vi "find_preamble2x1.vi"(0 "received \ntime symbol":cdb[](array[numeric]), 5 "FFT Size":u32, 7 "CP Length":u32, 9 "1st preamble":cdb[](array[numeric]), 11 "2nd preamble":cdb[](array[numeric])) -> (4 "OFDM Symbol":cdb[](array[numeric]))   [LabVIEW 2020]
uses:
  <vilib>/Analysis/2dsp.llb/Complex FFT.vi
  <vilib>/Analysis/baseanly.llb/Complex A x B.vi
  <vilib>/Analysis/NI_AALBase.lvlib
  <vilib>/Analysis/NI_AALPro.lvlib
panel:
  out "Waveform Chart 4":dbl[](graph)
  out "size(s)":i32
  out "Array":i32[](array[numeric])
  out "Waveform Chart 3":dbl[](graph)
  out "Channel Estimation":cdb[][](array[numeric])
  out "x-y":i32
  out "Waveform Chart 2":dbl[](graph)
  out "Waveform Chart":dbl[](graph)
  out "max value 2":dbl
  out "max value":dbl
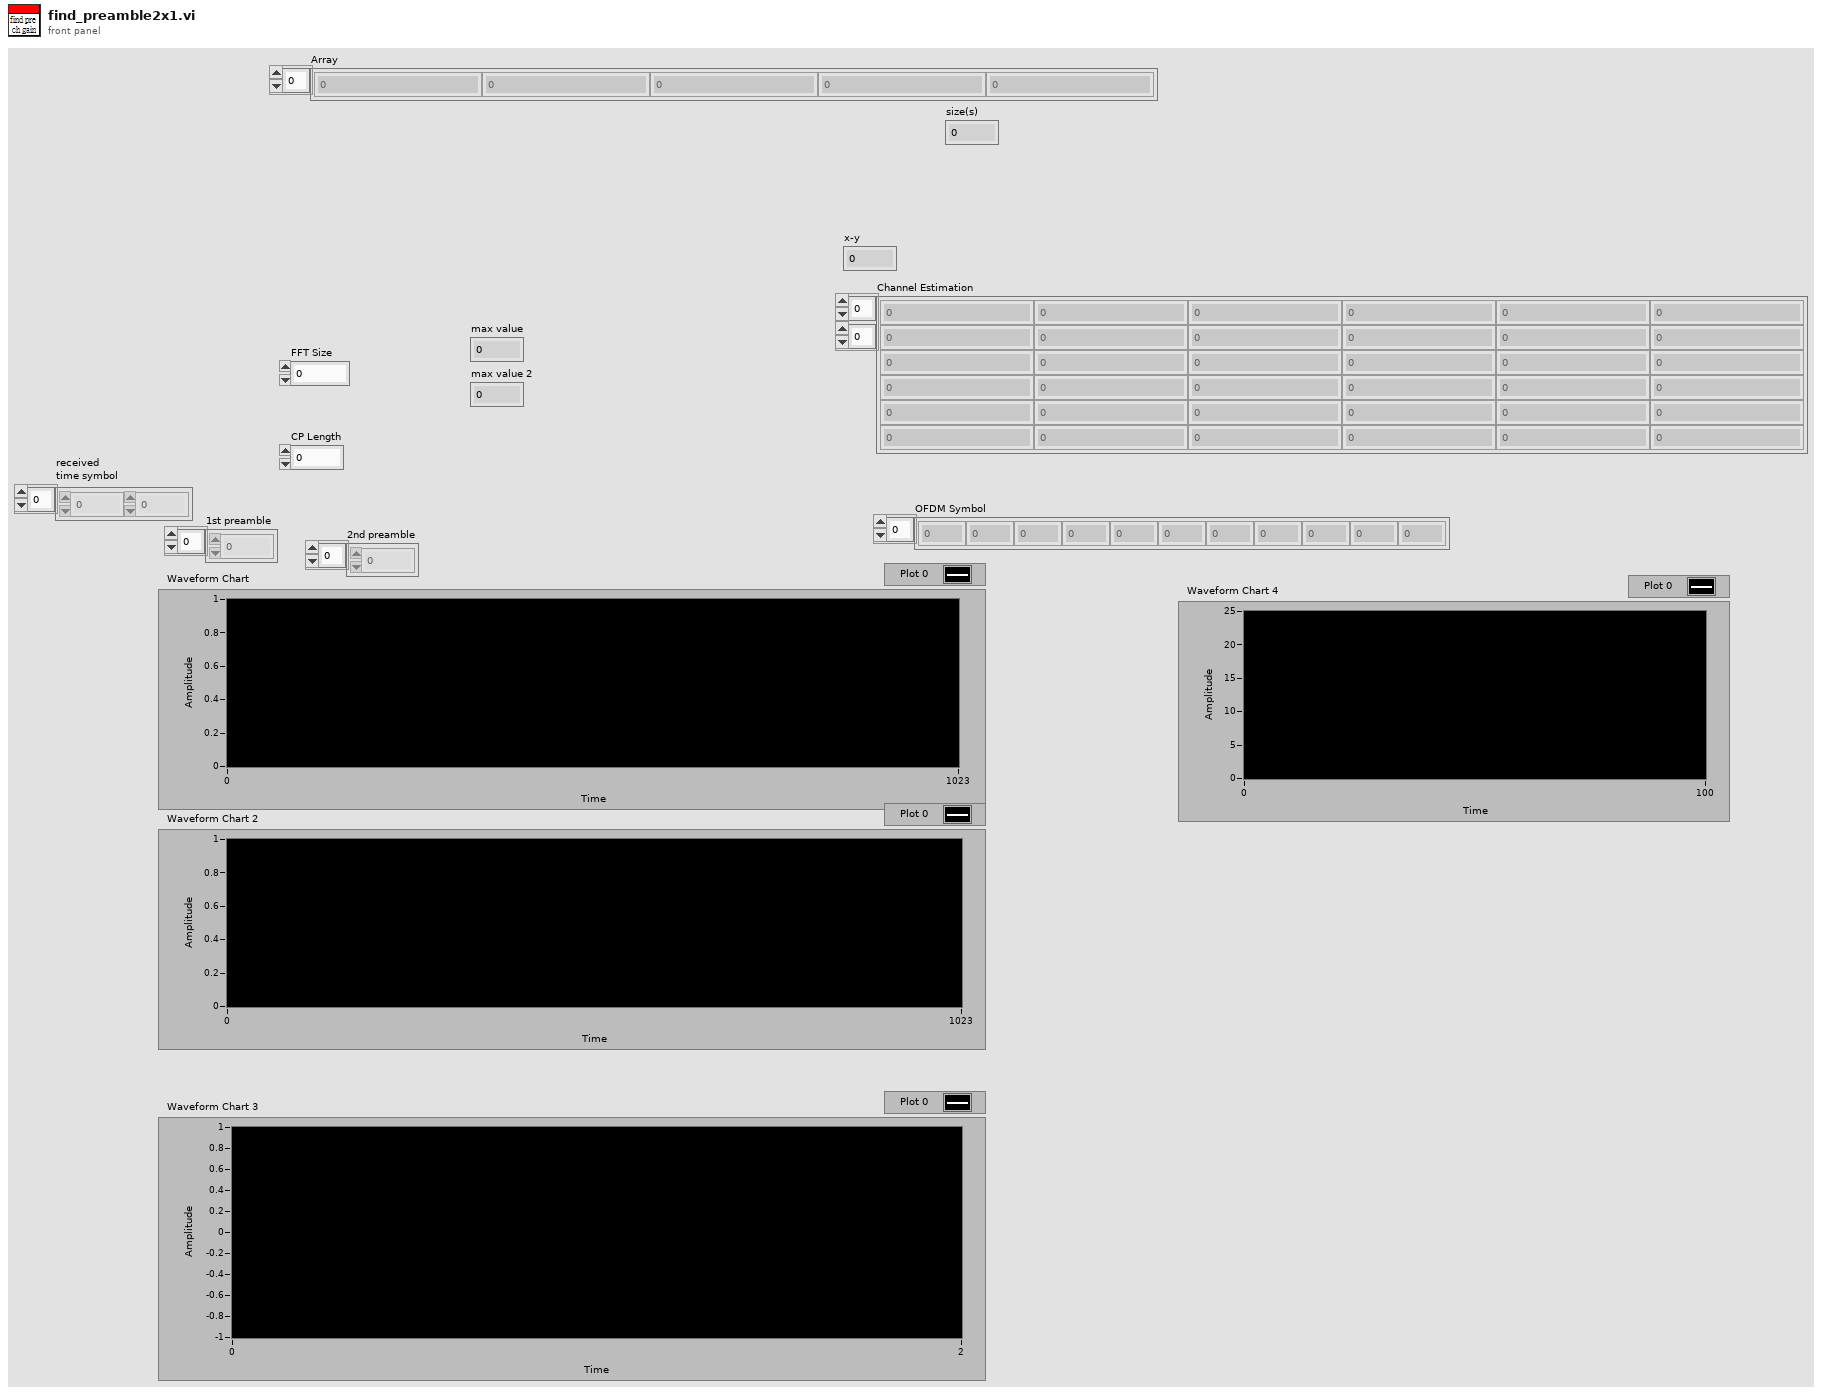
[diagram p1: front panel]
types:
  T1 = typedef "NI_Matrix.lvlib/ComplexMatrix.ctl" = cdb[][]
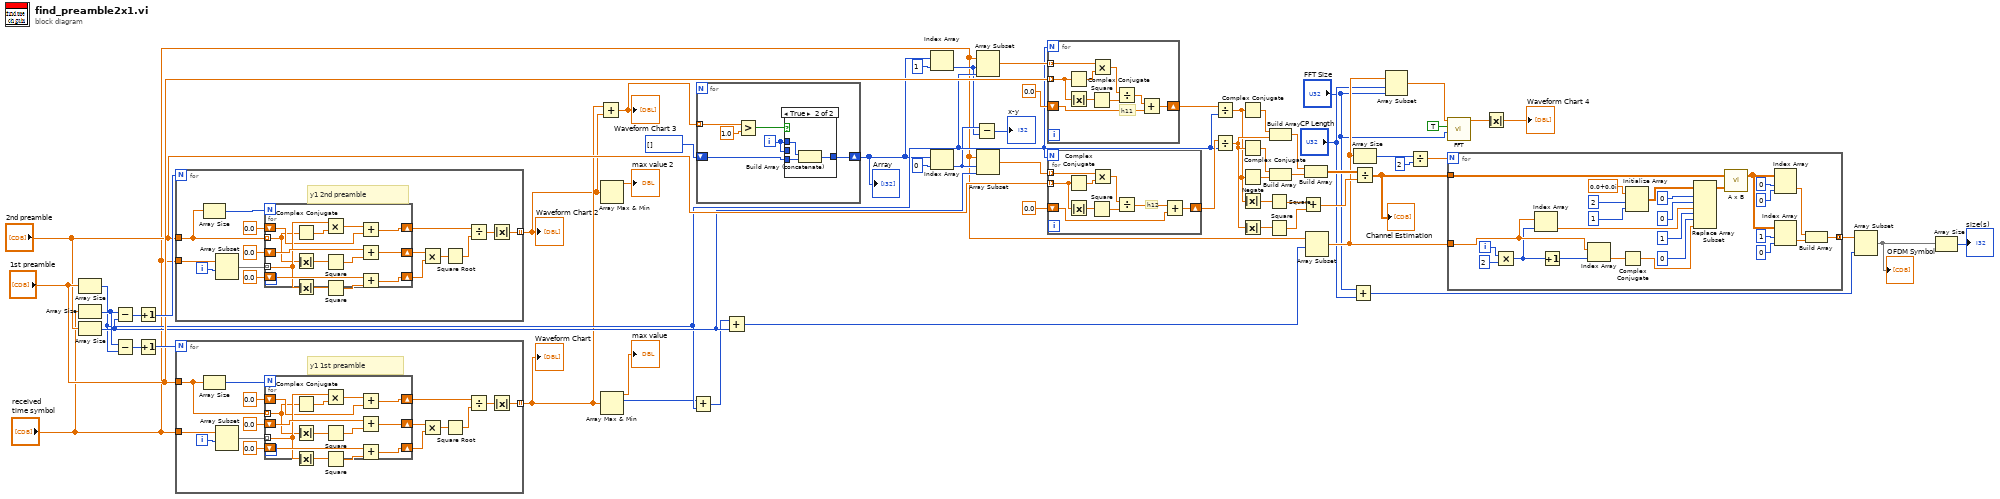
[diagram p0: block diagram]
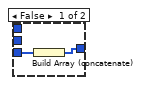
[diagram p2: hidden frame]
diagram:
  n1 = Array Size(array="1st preamble") -> (size(s)=w31:i32)
  n2 = Array Size(array="received \ntime symbol") -> (size(s)=w55:i32)
  n3 = Array Size(array="2nd preamble") -> (size(s)=w33:i32)
  n4 = Subtract(x=w55, y=w33) -> (x-y=w57:i32)
  n5 = Subtract(x=w55, y=w31) -> (x-y=w59:i32)
  n6 = Increment(x=w57) -> (x+1=w56:i32)
  n7 = Increment(x=w59) -> (x+1=w58:i32)
  n8 = for {
    N: w56 -> [_]
    tunnel: "2nd preamble" -> [w60]
    tunnel: "received \ntime symbol" -> [w61]
    tunnel: [w65] -> w19 mode=indexing
    i -> [w68]
    # "y1 2nd preamble"
    n9 = Array Size(array=w60) -> (size(s)=w74:i32)
    n10 = Array Subset(array=w61, index=w68) -> (w73:cdb[])  [unwired: 1 in]
    n11 = for {
      N: w74 -> [_]
      tunnel: w60 -> [w75] mode=indexing
      shift-right: [w85] -> w72
      shift-left: 0.0 -> [w87]
      shift-right: [w82] -> w71
      shift-left: 0.0 -> [w81]
      tunnel: w73 -> [w80] mode=indexing
      shift-right: [w76] -> w70
      shift-left: 0.0 -> [w77]
      n12 = Complex Conjugate(1:w75) -> (0:w79:cdb)
      n13 = Absolute Value(x=w75) -> (abs(x)=w88:dbl)
      n14 = Absolute Value(x=w80) -> (abs(x)=w84:dbl)
      n15 = Multiply(x=w80, y=w79) -> (x*y=w78:cdb)
      n16 = Square(x=w88) -> (x^2=w86:dbl)
      n17 = Square(x=w84) -> (x^2=w83:dbl)
      n18 = Add(x=w78, y=w77) -> (x+y=w76:cdb)
      n19 = Add(x=w87, y=w86) -> (x+y=w85:dbl)
      n20 = Add(x=w81, y=w83) -> (x+y=w82:dbl)
    }
    n21 = Multiply(x=w72, y=w71) -> (x*y=w67:dbl)
    n22 = Square Root(x=w67) -> (sqrt(x)=w66:dbl)
    n23 = Divide(x=w70, y=w66) -> (x/y=w69:cdb)
    n24 = Absolute Value(x=w69) -> (abs(x)=w65:dbl)
  }
  "Waveform Chart 2" <- w19
  n25 = for {
    N: w58 -> [_]
    tunnel: "received \ntime symbol" -> [w91]
    tunnel: "1st preamble" -> [w92]
    tunnel: [w90] -> w20 mode=indexing
    i -> [w89]
    # "y1 1st preamble"
    n26 = Array Size(array=w92) -> (size(s)=w93:i32)
    n27 = Array Subset(array=w91, index=w89) -> (w94:cdb[])  [unwired: 1 in]
    n28 = for {
      N: w93 -> [_]
      tunnel: w92 -> [w104] mode=indexing
      shift-right: [w114] -> w95
      shift-left: 0.0 -> [w116]
      shift-right: [w111] -> w96
      shift-left: 0.0 -> [w110]
      tunnel: w94 -> [w109] mode=indexing
      shift-right: [w105] -> w97
      shift-left: 0.0 -> [w106]
      n29 = Complex Conjugate(1:w104) -> (0:w108:cdb)
      n30 = Absolute Value(x=w104) -> (abs(x)=w117:dbl)
      n31 = Absolute Value(x=w109) -> (abs(x)=w113:dbl)
      n32 = Multiply(x=w109, y=w108) -> (x*y=w107:cdb)
      n33 = Square(x=w117) -> (x^2=w115:dbl)
      n34 = Square(x=w113) -> (x^2=w112:dbl)
      n35 = Add(x=w107, y=w106) -> (x+y=w105:cdb)
      n36 = Add(x=w116, y=w115) -> (x+y=w114:dbl)
      n37 = Add(x=w110, y=w112) -> (x+y=w111:dbl)
    }
    n38 = Multiply(x=w95, y=w96) -> (x*y=w99:dbl)
    n39 = Square Root(x=w99) -> (sqrt(x)=w100:dbl)
    n40 = Divide(x=w97, y=w100) -> (x/y=w98:cdb)
    n41 = Absolute Value(x=w98) -> (abs(x)=w90:dbl)
  }
  "Waveform Chart" <- w20
  n42 = Add(x=w20, y=w19) -> (x+y=w18:dbl[])
  "Waveform Chart 3" <- w18
  n43 = Array Max & Min(array=w19) -> (max value=→"max value 2":dbl)  [unwired: 3 out]
  n44 = Array Max & Min(array=w20) -> (max value=→"max value":dbl, max index (indices)=w25:i32)  [unwired: 2 out]
  n45 = Add(x=w25, y=w31) -> (x+y=w32:i32)
  n46 = for {
    tunnel: w18 -> [w123] mode=indexing
    shift-right: [w120] -> w15
    shift-left: i32[] [] -> [w119]
    i -> [w118]
    n47 = Greater?(x=w123, y=1.0) -> (0:w121:bool)
    n48 = case shown="True" w121 {
      tunnel: w118 -> [_ _]
      tunnel: [w125 w128] -> w120
      tunnel: w119 -> [w124 w126]
      tunnel: w118 -> [_ w127]
      frame False {
        n49 = Build Array (concatenate)(w124) -> (w125:i32[])
      }
      frame True {
        n50 = Build Array (concatenate)(w127, w126) -> (w128:i32[])
      }
    }
  }
  "Array" <- w15
  n51 = Add(x=w32, y=w33) -> (x+y=w30:i32)
  n52 = Index Array(array=w15, index=1) -> (element=w12:i32)
  n53 = Index Array(array=w15, index=0) -> (element=w13:i32)
  n54 = Subtract(x=w13, y=w12) -> (x-y=→"x-y":i32)
  n55 = Array Subset(array="received \ntime symbol", index=w12, length=w31) -> (w45:cdb[])
  n56 = Array Subset(array="received \ntime symbol", index=w13, length=w33) -> (w29:cdb[])
  n57 = for {
    N: w31 -> [_]
    shift-right: [w130] -> w51
    shift-left: 0.0 -> [w132]
    tunnel: w45 -> [w135] mode=indexing
    tunnel: "1st preamble" -> [w129] mode=indexing
    # "h11"
    n58 = Complex Conjugate(1:w129) -> (0:w137:cdb)
    n59 = Absolute Value(x=w129) -> (abs(x)=w136:dbl)
    n60 = Square(x=w136) -> (x^2=w133:dbl)
    n61 = Multiply(x=w135, y=w137) -> (x*y=w134:cdb)
    n62 = Divide(x=w134, y=w133) -> (x/y=w131:cdb)
    n63 = Add(x=w131, y=w132) -> (x+y=w130:cdb)
  }
  n64 = for {
    N: w31 -> [_]
    shift-right: [w140] -> w49
    shift-left: 0.0 -> [w142]
    tunnel: "2nd preamble" -> [w139] mode=indexing
    tunnel: w29 -> [w138] mode=indexing
    # "h12"
    n65 = Complex Conjugate(1:w139) -> (0:w146:cdb)
    n66 = Absolute Value(x=w139) -> (abs(x)=w145:dbl)
    n67 = Square(x=w145) -> (x^2=w143:dbl)
    n68 = Multiply(x=w138, y=w146) -> (x*y=w144:cdb)
    n69 = Divide(x=w144, y=w143) -> (x/y=w141:cdb)
    n70 = Add(x=w141, y=w142) -> (x+y=w140:cdb)
  }
  n71 = Divide(x=w51, y=w31) -> (x/y=w22:cdb)
  n72 = Divide(x=w49, y=w31) -> (x/y=w39:cdb)
  n73 = Complex Conjugate(1:w22) -> (0:w44:cdb)
  n74 = Complex Conjugate(1:w39) -> (0:w43:cdb)
  n75 = Negate(x=w22) -> (-x=w21:cdb)
  n76 = Absolute Value(x=w22) -> (abs(x)=w40:dbl)
  n77 = Absolute Value(x=w39) -> (abs(x)=w38:dbl)
  n78 = Square(x=w40) -> (x^2=w37:dbl)
  n79 = Square(x=w38) -> (x^2=w36:dbl)
  n80 = Build Array(w44, w39) -> (w42:cdb[])
  n81 = Build Array(w43, w21) -> (w41:cdb[])
  n82 = Add(x=w37, y=w36) -> (x+y=w35:dbl)
  n83 = Build Array(w42, w41) -> (w34:cdb[][])
  n84 = Array Subset(array="received \ntime symbol", index=w30) -> (w6:cdb[])  [unwired: 1 in]
  n85 = Add(x="FFT Size", y="CP Length") -> (x+y=w23:u32)
  n86 = Array Size(array=w6) -> (size(s)=w54:i32)
  n87 = Divide(x=w34, y=w35) -> (x/y=w8:cdb[][])
  "Channel Estimation" <- w8
  n88 = Array Subset "Array Subset"(array=w6, index="CP Length", length="FFT Size") -> (w3:cdb[])
  n89 = Divide(x=w54, y=2) -> (x/y=w52:dbl)
  n90 = call-poly <vilib>:"FFT.vi"("FFT size"="FFT Size", "shift?"=TRUE, "X"=w3) -> ("FFT {X}"=w2:cdb[])  [unwired: 7 in, 1 out]
  n91 = for {
    N: w52 -> [_]
    tunnel: w6 -> [w172]
    tunnel: [w154] -> w24 mode=concatenating
    tunnel: w8 -> [w166]
    i -> [w171]
    n92 = Multiply(x=w171, y=2) -> (x*y=w169:i32)
    n93 = Index Array(array=w172, index=w169) -> (element=w157:cdb)
    n94 = Increment(x=w169) -> (x+1=w168:i32)
    n95 = Index Array(array=w172, index=w168) -> (element=w167:cdb)
    n96 = Complex Conjugate(1:w167) -> (0:w156:cdb)
    n97 = Initialize Array(cdb 0.0+0.0i ("element"), 2 ("dimension size"), 1 ("dimension size")) -> (w162:cdb[][])
    n98 = Replace Array Subset(array=w162, new element #1=w157, index (row) #1=0 ("index (row)"), index (col) #1=0 ("disabled index (col)"), new element #2=w156, index (row) #2=1 ("index (row)"), index (col) #2=0 ("disabled index (col)")) -> (w155:cdb[][])
    n99 = call-poly <vilib>:"A x B.vi"("B"=w155, "A"=w166) -> ("A x B"=w153:T1)  [unwired: 1 out]
    n100 = Index Array(array=w153, index (row)=0, index (col)=0 ("disabled index (col)")) -> (element=w148:cdb)
    n101 = Index Array(array=w153, index (row)=1, index (col)=0 ("disabled index (col)")) -> (element=w147:cdb)
    n102 = Build Array(w148, w147) -> (w154:cdb[])
  }
  n103 = Absolute Value(x=w2) -> (abs(x)=→"Waveform Chart 4":dbl[])
  n104 = Array Subset(array=w24, length=w23) -> (w11:cdb[])  [unwired: 1 in]
  "OFDM Symbol" <- w11
  n105 = Array Size(array=w11) -> (size(s)=→"size(s)":i32)
